vi "Find Unreferenced Files.vi"() -> ()   [LabVIEW 2017, in "DocTools.lvlib"]
uses:
  DocTools.lvlib
panel:
  out "Unreferenced":i32
  out "Directory":i32
  out "Project":i32
  out "Tab Control":T1(tab)
  in  "Unreferenced Files":i32(listbox)
  in  "Project Files":i32(listbox)
  in  "Files in Directory":i32(listbox)
  in  "Project File":path=path "D:/Code/LabVIEW/_template/lv-doctools/lv-doctools.lvproj"
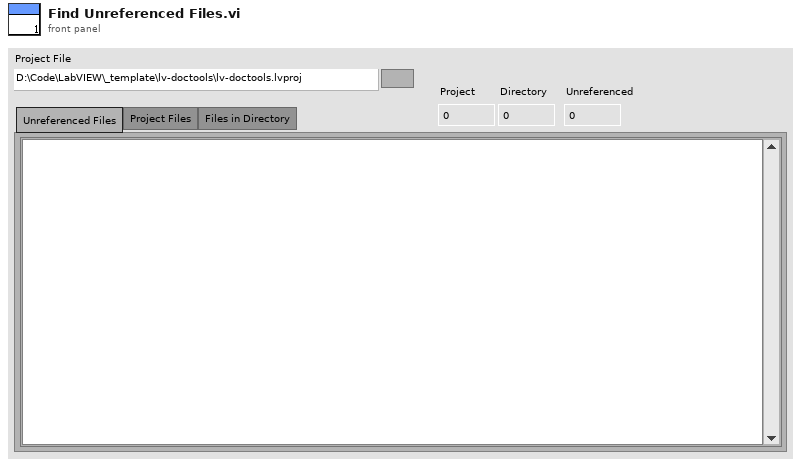
[diagram p1: front panel]
types:
  T1 = enum32{"Unreferenced Files", "Project Files", "Files in Directory"}
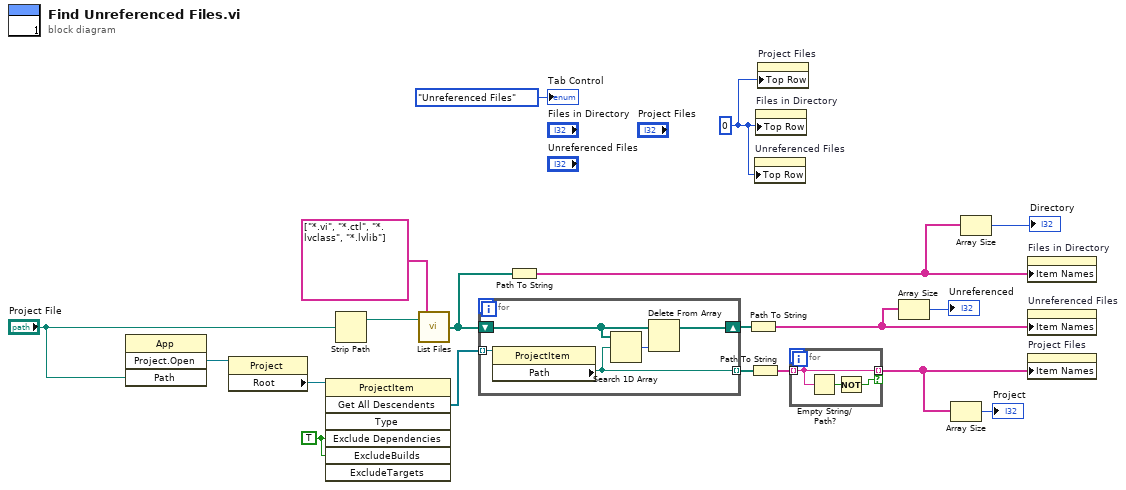
[diagram p0: block diagram]
diagram:
  w8 = 0
  w14 = TRUE ("ExcludeDependencies")
  n1 = invoke class="App" method="Project.Open"("Path"="Project File") -> ("Project:Open"=w16:refnum<vi>)  [unwired: 3 in, 3 out]
  n2 = property class="Project"(reference=w16) -> ("Root"=w15:refnum<vi>)  [unwired: 1 in, 2 out]
  n3 = invoke class="ProjectItem" method="Get All Descendents"(reference=w15, "Exclude Dependencies"=w14, "ExcludeBuilds"=w14) -> ("All Descendents"=w13:refnum<vi>[])  [unwired: 4 in, 6 out]
  n4 = Strip Path(path="Project File") -> (stripped path=w19:path)  [unwired: 1 out]
  n5 = call "List Files.vi"("File Pattern[] (e.g. *.vi)"=string[] ["*.vi", "*.ctl", "*.lvclass", "*.lvlib"], "Root Path"=w19) -> ("File Path[]"=w11:path[])
  n6 = for {
    tunnel: w13 -> [w24] mode=indexing
    shift-right: [w21] -> w12
    shift-left: w11 -> [w23]
    tunnel: [w20] -> w10 mode=indexing
    n7 = property class="ProjectItem"(reference=w24) -> ("Path"=w20:path)  [unwired: 1 in, 2 out]
    n8 = Search 1D Array(1D array=w23, element=w20) -> (index of element=w22:i32)  [unwired: 1 in]
    n9 = Delete From Array(array=w23, index=w22) -> (array with subset deleted=w21:path[])  [unwired: 1 in, 1 out]
  }
  n10 = Path To String(path=w11) -> (string=w4:string[])
  n11 = Path To String(path=w12) -> (string=w1:string[])
  n12 = Path To String(path=w10) -> (string=w7:string[])
  n13 = property on="Unreferenced Files" class="LstBox (strict)"("Top Row"=w8) -> ()  [unwired: 2 in, 2 out]
  n14 = property on="Files in Directory" class="LstBox (strict)"("Top Row"=w8) -> ()  [unwired: 2 in, 2 out]
  n15 = property on="Project Files" class="LstBox (strict)"("Top Row"=w8) -> ()  [unwired: 2 in, 2 out]
  n16 = for {
    tunnel: w7 -> [w26] mode=indexing
    tunnel: [w26] -> w5 mode=indexing if=w25
    n17 = Empty String/Path?(string/path=w26) -> (empty?=w27:bool)
    n18 = Not(x=w27) -> (.not. x?=w25:bool)
  }
  n19 = Array Size(array=w1) -> (size(s)=→"Unreferenced":i32)
  n20 = Array Size(array=w5) -> (size(s)=→"Project":i32)
  n21 = Array Size(array=w4) -> (size(s)=→"Directory":i32)
  n22 = property on="Files in Directory" class="LstBox (strict)"("Item Names"=w4) -> ()  [unwired: 2 in, 2 out]
  n23 = property on="Unreferenced Files" class="LstBox (strict)"("Item Names"=w1) -> ()  [unwired: 2 in, 2 out]
  n24 = property on="Project Files" class="LstBox (strict)"("Item Names"=w5) -> ()  [unwired: 2 in, 2 out]
  "Tab Control" <- T1."Unreferenced Files" ("Tab Control")
